vi "brc_daq_disconnect_module.vi"(0 "index":i32, 5 "error in (no error)":errorcluster, 6 "mHandle":i32) -> (19 "error out":errorcluster)   [LabVIEW 2019, in "BRC-DAQ.lvlib"]
uses:
  BRC-DAQ.lvlib
panel:
  out "return_value":i32
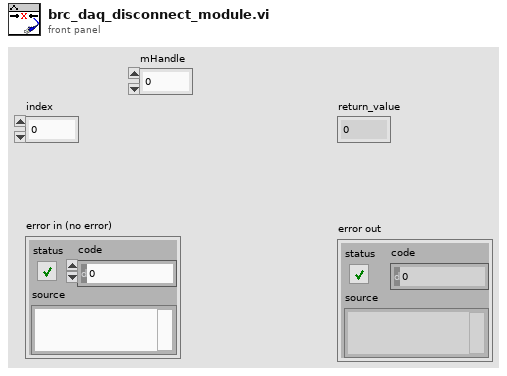
[diagram p1: front panel]
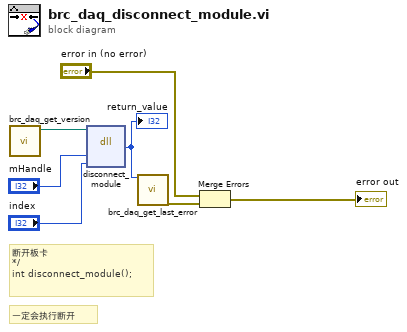
[diagram p0: block diagram]
diagram:
  # "断开板卡\n*/\nint disconnect_module();"
  # "一定会执行断开"
  n1 = call "brc_daq_get_version.vi"() -> ("dll path"=w1:path)  [unwired: 11 in]
  n2 = dll-call lib="E:/01 BRC project/04BRC-daq/04 Drive/DAQ-x64/DLL/brc_daq_sdk.dll" fn="disconnect_module"(path in=w1, "mHandle"="mHandle", "index"="index") -> ("return type"=w4:i32)  [unwired: 4 in, 2 out]
  "return_value" <- w4
  n3 = call "brc_daq_get_last_error.vi"("return_value"=w4) -> ("error out"=w3:errorcluster)  [unwired: 18 in]
  n4 = Merge Errors("error in (no error)", w3) -> (→"error out":errorcluster)
